vi "Init_Camera.vi"(10 "Camera IP":string="10.4.49.11") -> (3 "CameraDevRef Out":T1)   [LabVIEW 2011]
uses:
  <vilib>/Rock Robotics/WPI/Camera/WPI_CameraImageSize.ctl
  <vilib>/Rock Robotics/WPI/Camera/WPI_CameraDevRef.ctl
  <vilib>/Rock Robotics/WPI/Camera/WPI_CameraWhite Balance Values.ctl
  <vilib>/Rock Robotics/WPI/Camera/WPI_CameraExposure Values.ctl
  <vilib>/Rock Robotics/WPI/Camera/WPI_CameraFrameRate.ctl
panel:
  in  "Image Size":T2=enum."320x240"
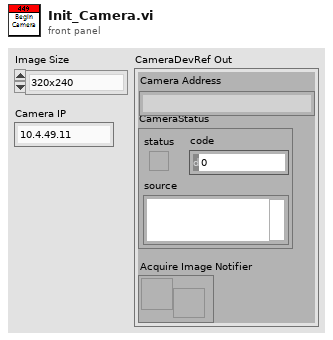
[diagram p1: front panel]
types:
  T1 = typedef "WPI_CameraDevRef.ctl" = cluster{"Camera Address":string, "CameraStatus":errorcluster, "Acquire Image Notifier":refnum<notifier>}
  T2 = typedef "WPI_CameraImageSize.ctl" = enum16{"640x480", "320x240", "160x120"}
  T3 = typedef "WPI_CameraFrameRate.ctl" = u32
  T4 = typedef "WPI_CameraExposure Values.ctl" = enum16{"Auto", "Flicker-free 50 Hz", "Flicker-free 60 Hz", "Hold current"}
  T5 = typedef "WPI_CameraWhite Balance Values.ctl" = enum16{"Auto", "Fixed indoor", "Fixed outdoor 1", "Fixed outdoor 2", "Fixed fluorescent 1", "Fixed fluorescent 2", "Hold current"}
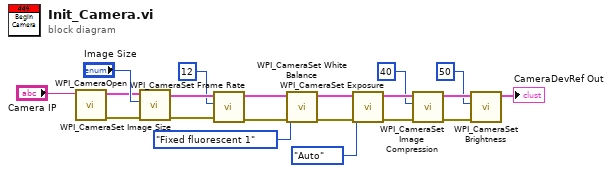
[diagram p0: block diagram]
diagram:
  n1 = call <vilib>:"WPI_CameraOpen.vi"("Camera Address"="Camera IP") -> ("error out"=w11:errorcluster, "CameraDevRef"=w19:T1)  [unwired: 9 in]
  n2 = call <vilib>:"WPI_CameraSet Image Size.vi"("error in (no error)"=w11, "Image Size"="Image Size", "CameraDevRef"=w19) -> ("error out"=w10:errorcluster, "CameraDevRef Out"=w18:T1)  [unwired: 7 in]
  n3 = call <vilib>:"WPI_CameraSet Frame Rate.vi"("error in (no error)"=w10, "Frame Rate (fps)"=T3 12, "CameraDevRef"=w18) -> ("error out"=w9:errorcluster, "CameraDevRef Out"=w17:T1)  [unwired: 7 in]
  n4 = call <vilib>:"WPI_CameraSet White Balance.vi"("error in (no error)"=w9, "White Balance"=WPI_CameraWhite_Balance_Values."Fixed fluorescent 1", "CameraDevRef"=w17) -> ("error out"=w8:errorcluster, "CameraDevRef Out"=w15:T1)  [unwired: 7 in]
  n5 = call <vilib>:"WPI_CameraSet Exposure.vi"("error in (no error)"=w8, "Exposure"=WPI_CameraExposure_Values."Auto", "CameraDevRef"=w15) -> ("error out"=w13:errorcluster, "CameraDevRef Out"=w12:T1)  [unwired: 7 in]
  n6 = call <vilib>:"WPI_CameraSet Image Compression.vi"("error in (no error)"=w13, "Compression"=40, "CameraDevRef"=w12) -> ("error out"=w5:errorcluster, "CameraDevRef Out"=w4:T1)  [unwired: 7 in]
  n7 = call <vilib>:"WPI_CameraSet Brightness.vi"("error in (no error)"=w5, "Brightness"=50, "CameraDevRef"=w4) -> ("CameraDevRef Out"=→"CameraDevRef Out":T1)  [unwired: 7 in, 1 out]
